vi "Memory.Pointer.Error Handling.Out of Range.vi"(5 "parameter":T1, 7 "source vi name":string, 8 "error in (no error)":errorcluster, 9 "min":i64 format="%d bytes", 10 "value":i64 format="%d bytes", 11 "max":i64 format="%d bytes") -> (0 "error out":errorcluster)   [LabVIEW 2016, in "LabVIEW Memory Manager.lvlib" / "Memory.Pointer.lvclass"]
uses:
  Memory.Pointer.lvclass
  Typedefs/Memory.Pointer.Parameters.ctl
  Typedefs/Memory.Pointer.Error Codes.ctl
  RT Errors/VIs/Deterministic Errors.New Error Cluster (256B).vi
  Memory.Globals.vi
  RT Errors/Deterministic Error Builder.lvlib
  LabVIEW Memory Manager.lvlib
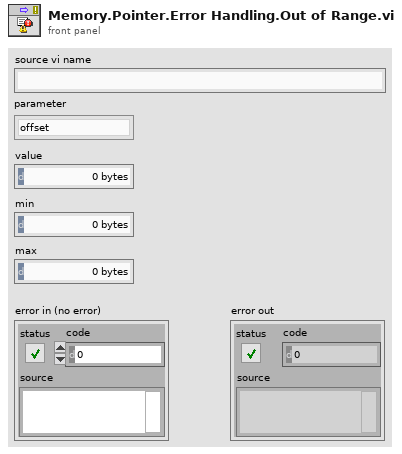
[diagram p1: front panel]
types:
  T1 = typedef "LabVIEW Memory Manager.lvlib/Memory.Pointer.lvclass/Memory.Pointer.Parameters.ctl" = enum16{"offset", "length", "size", "subset"}
  T2 = typedef "LabVIEW Memory Manager.lvlib/Memory.Pointer.lvclass/Memory.Pointer.Error Codes.ctl" = enum16{"Out of range"}
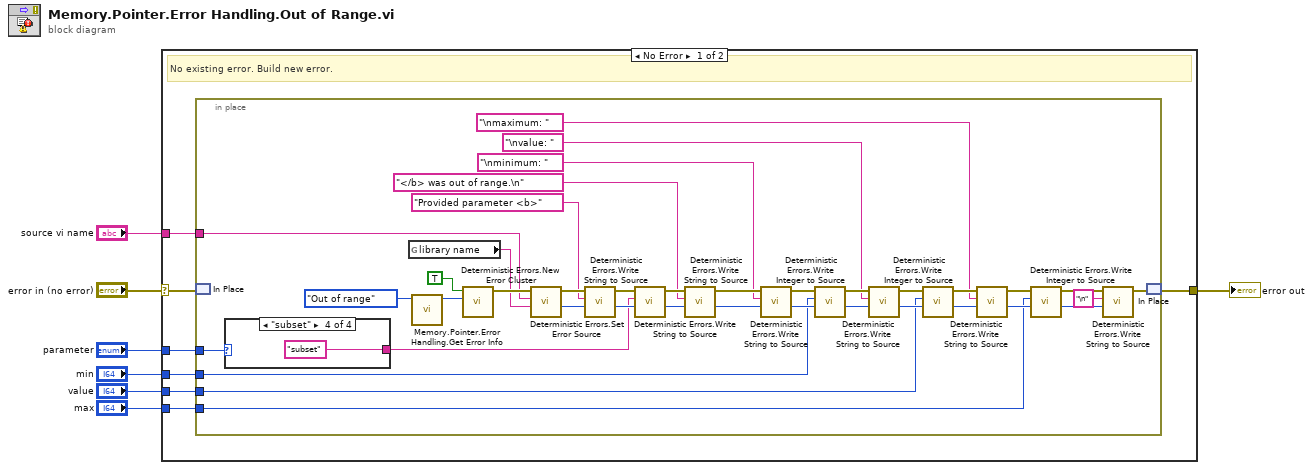
[diagram p0: block diagram]
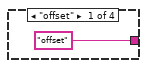
[diagram p2: hidden frame]
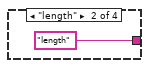
[diagram p3: hidden frame]
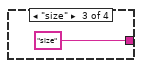
[diagram p4: hidden frame]
diagram:
  n1 = case shown="No Error" "error in (no error)" {
    selector: "error in (no error)" -> [w13 w57]
    tunnel: [w14 w57] -> w2
    tunnel: "value" -> [w11 _]
    tunnel: "min" -> [w10 _]
    tunnel: "max" -> [w9 _]
    tunnel: "source vi name" -> [w12 _]
    tunnel: "parameter" -> [w8 _]
    frame No Error {
      # "No existing error. Build new error."
      n2 = in-place {
        in-place-border: w12 -> [w49]
        in-place-border: w11 -> [w40]
        in-place-border: w10 -> [w18]
        in-place-border: w9 -> [w33]
        in-place-border: w8 -> [w16]
        n3 = in-place-match #1(w13) -> ()  [unwired: 1 out]
        n4 = case shown="\"subset\"" w16 {
          tunnel: ["offset" ("string") "length" ("string") "size" ("string") "subset" ("string")] -> w15
          frame "offset" {
          }
          frame "length" {
          }
          frame "size" {
          }
          frame "subset" {
          }
        }
        n5 = global read "Memory.Globals.vi" "library name"() -> (w27:string)
        n6 = call "Memory.Pointer.Error Handling.Get Error Info.vi"("error"=Memory.Pointer.Error_Codes."Out of range" ("error code")) -> ("code"=w50:i32)  [unwired: 9 in, 1 out]
        n7 = call-poly "Deterministic Errors.New Error Cluster.vi"("code (0)"=w50, "status (F)"=TRUE) -> ("error out"=w52:errorcluster)  [unwired: 9 in]
        n8 = call "Deterministic Errors.Set Error Source.vi"("library name (\"\")"=w27, "vi name"=w49, "error in"=w52) -> ("new offset"=w34:i32, "error out"=w35:errorcluster)  [unwired: 7 in]
        n9 = call "Deterministic Errors.Write String to Source.vi"("offset (0)"=w34, "string"="Provided parameter <b>", "error in"=w35) -> ("new offset"=w23:i32, "error out"=w25:errorcluster)  [unwired: 7 in]
        n10 = call "Deterministic Errors.Write String to Source.vi"("offset (0)"=w23, "string"=w15, "error in"=w25) -> ("new offset"=w22:i32, "error out"=w24:errorcluster)  [unwired: 7 in]
        n11 = call "Deterministic Errors.Write String to Source.vi"("offset (0)"=w22, "string"="</b> was out of range.\n", "error in"=w24) -> ("new offset"=w21:i32, "error out"=w20:errorcluster)  [unwired: 7 in]
        n12 = call "Deterministic Errors.Write String to Source.vi"("offset (0)"=w21, "string"="\nminimum: ", "error in"=w20) -> ("new offset"=w45:i32, "error out"=w48:errorcluster)  [unwired: 7 in]
        n13 = call "Deterministic Errors.Write Integer to Source.vi"("offset (0)"=w45, "value"=w18, "error in"=w48) -> ("new offset"=w46:i32, "error out"=w47:errorcluster)  [unwired: 7 in]
        n14 = call "Deterministic Errors.Write String to Source.vi"("offset (0)"=w46, "string"="\nvalue: ", "error in"=w47) -> ("new offset"=w41:i32, "error out"=w42:errorcluster)  [unwired: 7 in]
        n15 = call "Deterministic Errors.Write Integer to Source.vi"("offset (0)"=w41, "value"=w40, "error in"=w42) -> ("new offset"=w38:i32, "error out"=w39:errorcluster)  [unwired: 7 in]
        n16 = call "Deterministic Errors.Write String to Source.vi"("offset (0)"=w38, "string"="\nmaximum: ", "error in"=w39) -> ("new offset"=w36:i32, "error out"=w37:errorcluster)  [unwired: 7 in]
        n17 = call "Deterministic Errors.Write Integer to Source.vi"("offset (0)"=w36, "value"=w33, "error in"=w37) -> ("new offset"=w28:i32, "error out"=w31:errorcluster)  [unwired: 7 in]
        n18 = call "Deterministic Errors.Write String to Source.vi"("offset (0)"=w28, "string"="\n", "error in"=w31) -> ("error out"=w30:errorcluster)  [unwired: 7 in, 1 out]
        n19 = in-place-match #1(w30) -> (w14:errorcluster)
      }
    }
    frame Error {
      # "Incoming error. Pass through."
    }
  }
  "error out" <- w2
